vi "SolonoidAccess.vi"() -> ()   [LabVIEW 2011]
panel:
  in  "stop":bool
  in  "MG17Motor":refnum<k7>(container)
  in  "Port":u16=5020
  in  "IP":string="127.0.0.1"
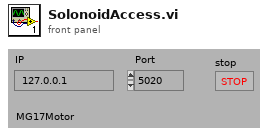
[diagram p1: front panel]
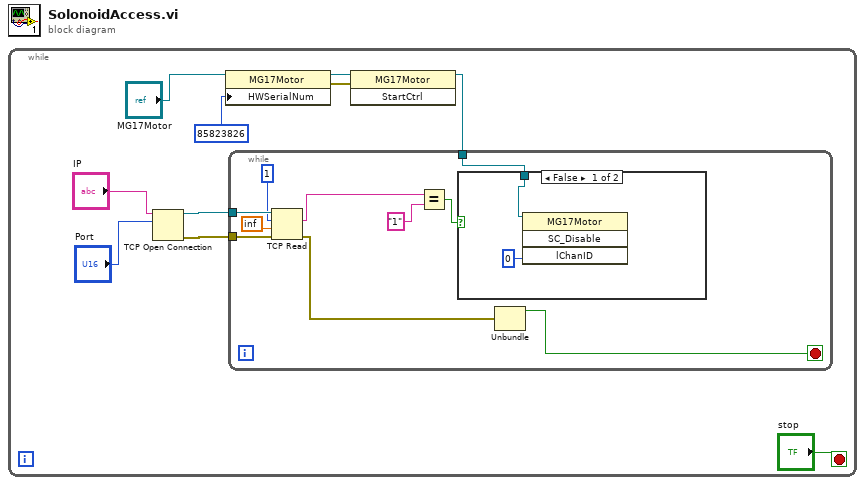
[diagram p0: block diagram]
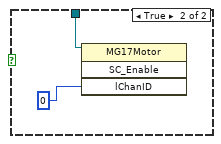
[diagram p2: hidden frame]
diagram:
  n1 = while {
    stop <- "stop" stop-if-true
    n2 = TCP Open Connection(address="IP", remote port or service name="Port") -> (connection ID=w10:refnum<k5>, error out=w9:errorcluster)  [unwired: 3 in]
    n3 = property class="MG17Motor"(reference="MG17Motor", "HWSerialNum"=85823826 ("lChanID")) -> (reference out=w5:refnum<k7>, error out=w4:errorcluster)  [unwired: 1 in]
    n4 = invoke class="MG17Motor" method="StartCtrl"(reference=w5, error in=w4) -> (reference out=w2:refnum<k7>)  [unwired: 1 in, 2 out]
    n5 = while {
      tunnel: w10 -> [w20]
      tunnel: w9 -> [w19]
      tunnel: w2 -> [w13]
      stop <- w16 stop-if-true
      n6 = TCP Read(connection ID=w20, bytes to read=1, error in (no error)=w19, 9:inf) -> (data out=w14:string, error out=w17:errorcluster)  [unwired: 1 in, 1 out]
      n7 = Equal?(x=w14, y="1") -> (x = y?=w12:bool)
      n8 = case shown="False" w12 {
        tunnel: w13 -> [w21 w24]
        frame False {
          n9 = invoke class="MG17Motor" method="SC_Disable"(reference=w21, "lChanID"=0) -> ()  [unwired: 2 in, 4 out]
        }
        frame True {
          n10 = invoke class="MG17Motor" method="SC_Enable"(reference=w24, "lChanID"=0) -> ()  [unwired: 2 in, 4 out]
        }
      }
      n11 = Unbundle(w17) -> ("status"=w16:bool)  [unwired: 2 out]
    }
  }
